vi "average fifo data.vi"(7 "Interleaved Data":i16[](array[numeric]), 17 "Samples":i32=1000, 18 "Acc":i32=200, 19 "error in (no error)":errorcluster) -> (6 "CD_signals":waveform(dbl), 8 "Avg Scan":dbl[](graph), 14 "error out (no error)":errorcluster)   [LabVIEW 2015, in "io runtime.lvclass"]
uses:
  io runtime.lvclass
  <vilib>/Analysis/NI_AALBase.lvlib
  <vilib>/Analysis/baseanly.llb/Mean (DBL).vi
panel:
  in  "Channels":i32=4
  out "Avg Scan+1":dbl[](graph)
  out "Low DC":dbl
  out "DC":dbl
  out "First 5000":i16[](graph)
  out "Process Time":u32
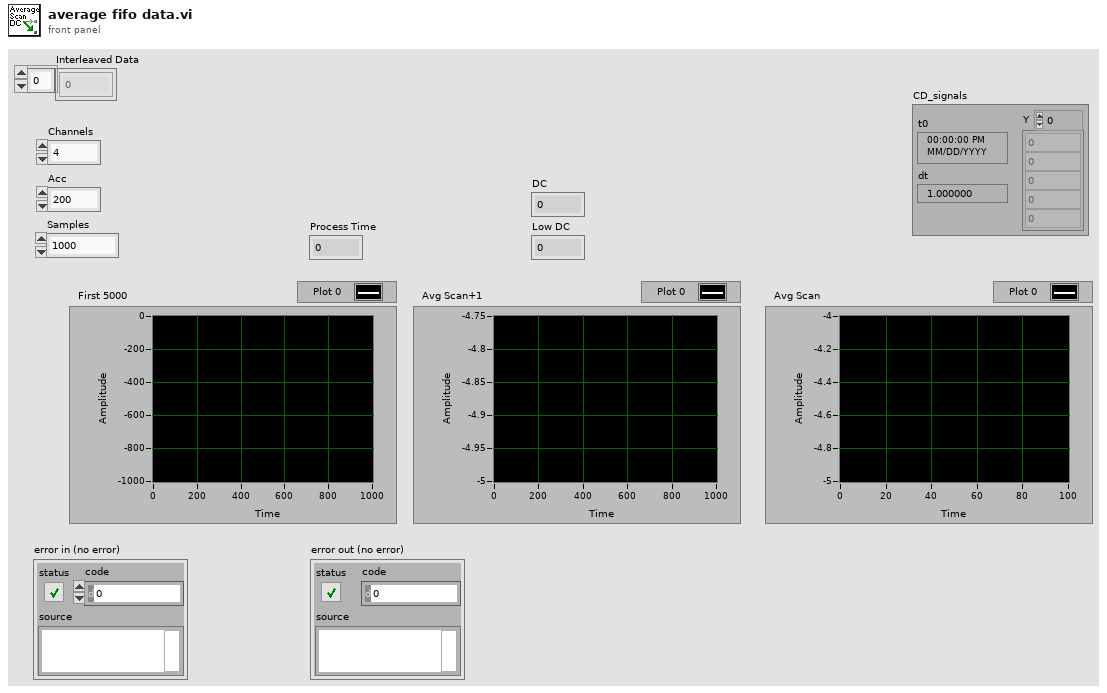
[diagram p1: front panel]
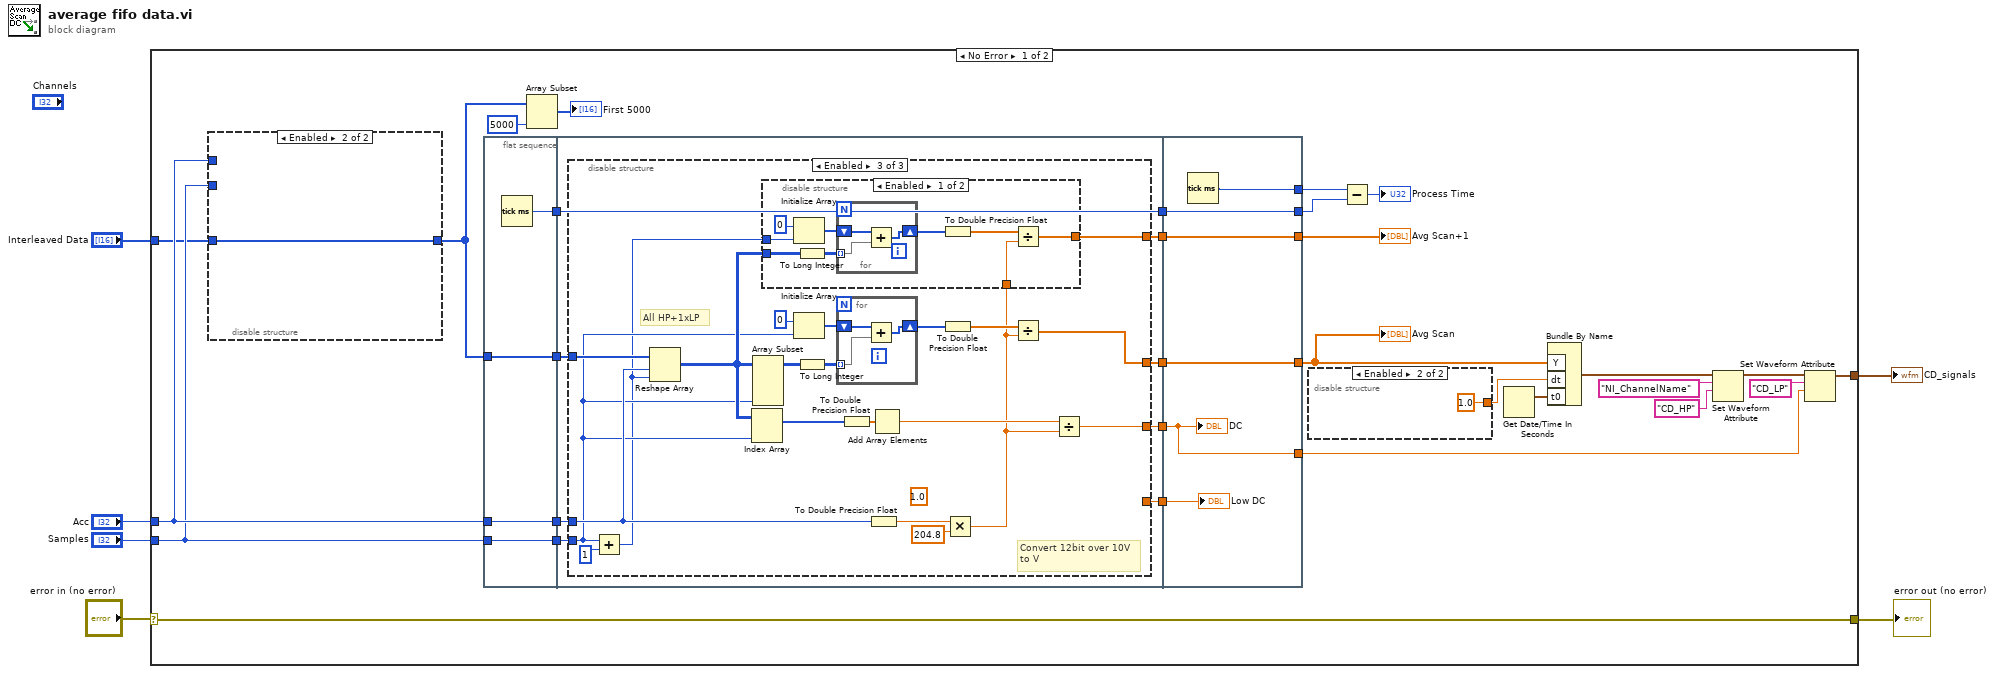
[diagram p0: block diagram]
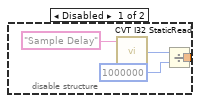
[diagram p2: hidden frame]
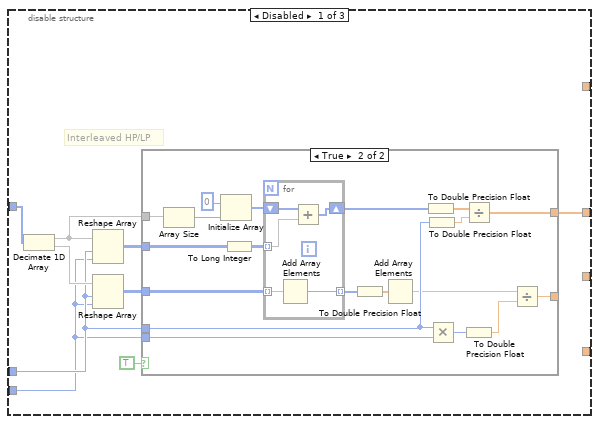
[diagram p3: hidden frame]
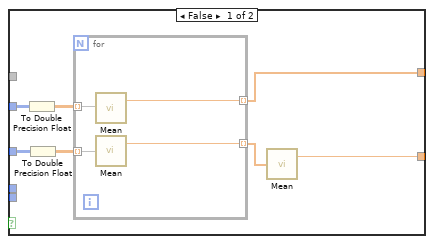
[diagram p4: hidden frame]
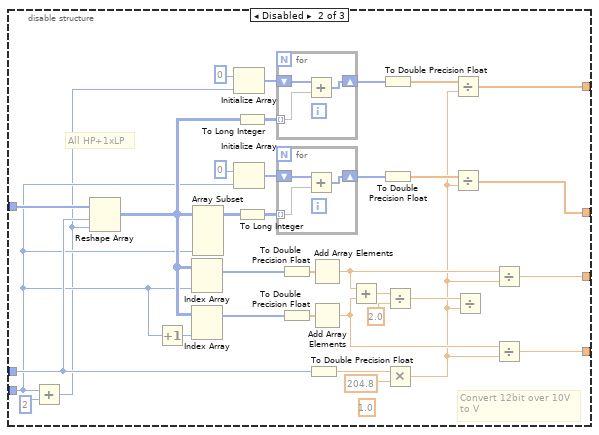
[diagram p5: hidden frame]
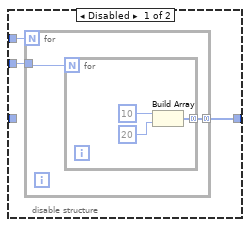
[diagram p7: hidden frame]
diagram:
  n1 = case shown="No Error" "error in (no error)" {
    selector: "error in (no error)" -> [w33 w189]
    tunnel: "Acc" -> [w36 _]
    tunnel: "Samples" -> [w35 _]
    tunnel: "Interleaved Data" -> [w34 _]
    tunnel: [w33 w189] -> w2
    tunnel: [w7 _] -> w1
    frame No Error {
      n2 = disable-structure shown="Enabled" {
        disable-tunnel: [w182 w188] -> w19
        disable-tunnel: w36 -> [w181 _]
        disable-tunnel: w35 -> [w180 _]
        disable-tunnel: w34 -> [_ w188]
        frame Disabled {
          n3 = for {
            N: w181 -> [_]
            tunnel: [w184] -> w182 mode=concatenating
            tunnel: w180 -> [w183]
            n4 = for {
              N: w183 -> [_]
              tunnel: [w185] -> w184 mode=concatenating
              n5 = Build Array(10, 20) -> (w185:i32[])
            }
          }
        }
        frame Enabled {
        }
      }
      n6 = flat-sequence {
        tunnel: w35 -> [w43]
        tunnel: w36 -> [w44]
        tunnel: w19 -> [w45]
        tunnel: [w45] -> w27
        tunnel: [w44] -> w26
        tunnel: [w43] -> w25
        tunnel: [w42] -> w20
        tunnel: w27 -> [w53]
        tunnel: w26 -> [w52]
        tunnel: w25 -> [w51]
        tunnel: [w50] -> w24
        tunnel: [w49] -> w21
        tunnel: w20 -> [w49]
        tunnel: [w48] -> w15
        tunnel: [w47] -> w14
        tunnel: [w46] -> w13
        tunnel: [w174] -> w8
        tunnel: [w175] -> w12
        tunnel: w24 -> [w175]
        tunnel: [w179] -> w22
        tunnel: [w178] -> w11
        tunnel: w21 -> [w178]
        tunnel: [w177] -> w16
        tunnel: w15 -> [w177]
        tunnel: w14 -> [w174]
        tunnel: w13 -> [w176]
        frame #0 {
          n7 = Tick Count (ms)() -> (millisecond timer value=w42:u32)
        }
        frame #1 {
          n8 = disable-structure shown="Enabled" {
            disable-tunnel: w53 -> [w58 w123 w150]
            disable-tunnel: w52 -> [w57 w122 w149]
            disable-tunnel: w51 -> [w56 w103 w142]
            disable-tunnel: [w55 w121 w148] -> w50
            disable-tunnel: [_ w104 w143] -> w48
            disable-tunnel: [_ w100 w140] -> w47
            disable-tunnel: [_ w99 _] -> w46
            frame Disabled {
              # "Interleaved HP/LP"
              n9 = Decimate 1D Array(w58) -> (w59:i16[], w62:i16[])
              n10 = Reshape Array(w59, w57, w56) -> (w61:i16[][])
              n11 = Reshape Array(w62, w57, w56) -> (w60:i16[][])
              n12 = case shown="True" TRUE {
                tunnel: w57 -> [_ w92]
                tunnel: w61 -> [w69 w91]
                tunnel: w60 -> [w68 w90]
                tunnel: w59 -> [_ w84]
                tunnel: [w63 w83] -> _
                tunnel: w56 -> [_ w77]
                tunnel: [w67 w76] -> w55
                frame False {
                  n13 = To Double Precision Float(number=w69) -> (double precision float=w66:dbl[][])
                  n14 = To Double Precision Float(number=w68) -> (double precision float=w65:dbl[][])
                  n15 = for {
                    tunnel: w66 -> [w73] mode=indexing
                    tunnel: w65 -> [w71] mode=indexing
                    tunnel: [w72] -> w67 mode=indexing
                    tunnel: [w70] -> w64 mode=indexing
                    n16 = call-poly <vilib>:"Mean.vi"("X"=w73) -> ("mean"=w72:dbl)  [unwired: 1 out]
                    n17 = call-poly <vilib>:"Mean.vi"("X"=w71) -> ("mean"=w70:dbl)  [unwired: 1 out]
                  }
                  n18 = call-poly <vilib>:"Mean.vi"("X"=w64) -> ("mean"=w63:dbl)  [unwired: 1 out]
                }
                frame True {
                  n19 = Array Size(array=w84) -> (size(s)=w85:i32)
                  n20 = Initialize Array(0, w85) -> (w87:i32[])
                  n21 = To Long Integer(number=w91) -> (32bit integer=w78:i32[][])
                  n22 = for {
                    tunnel: w78 -> [w96] mode=indexing
                    shift-right: [w97] -> w89
                    shift-left: w87 -> [w95]
                    tunnel: w90 -> [w94] mode=indexing
                    tunnel: [w93] -> w81 mode=indexing
                    n23 = Add Array Elements(numeric array=w94) -> (sum=w93:i16)
                    n24 = Add(x=w95, y=w96) -> (x+y=w97:i32[])
                  }
                  n25 = To Double Precision Float(number=w81) -> (double precision float=w80:dbl[])
                  n26 = Add Array Elements(numeric array=w80) -> (sum=w79:dbl)
                  n27 = To Double Precision Float(number=w89) -> (double precision float=w88:dbl[])
                  n28 = To Double Precision Float(number=w92) -> (double precision float=w82:dbl)
                  n29 = Multiply(x=w92, y=w77) -> (x*y=w75:i32)
                  n30 = Divide(x=w88, y=w82) -> (x/y=w76:dbl[])
                  n31 = To Double Precision Float(number=w75) -> (double precision float=w74:dbl)
                  n32 = Divide(x=w79, y=w74) -> (x/y=w83:dbl)
                }
              }
            }
            frame Disabled {
              (unwired) 1.0 ("y")
              # "Convert 12bit over 10V\nto V"
              # "All HP+1xLP"
              n33 = Add(x=w103, y=2) -> (x+y=w102:i32)
              n34 = Reshape Array(w123, w122, w102) -> (w106:i16[][])
              n35 = Increment(x=w103) -> (x+1=w114:i32)
              n36 = Index Array(array=w106, index (col)=w103) -> (element=w124:i16[])  [unwired: 1 in]
              n37 = Index Array(array=w106, index (col)=w114) -> (element=w119:i16[])  [unwired: 1 in]
              n38 = Array Subset(array=w106, length (col)=w103) -> (w125:i16[][])  [unwired: 3 in]
              n39 = Initialize Array(0, w102) -> (w108:i32[])
              n40 = Initialize Array(0, w103) -> (w129:i32[])
              n41 = To Long Integer(number=w106) -> (32bit integer=w110:i32[][])
              n42 = To Long Integer(number=w125) -> (32bit integer=w126:i32[][])
              n43 = for {
                tunnel: w110 -> [w133] mode=indexing
                shift-right: [w134] -> w107
                shift-left: w108 -> [w132]
                n44 = Add(x=w132, y=w133) -> (x+y=w134:i32[])
              }
              n45 = for {
                tunnel: w126 -> [w136] mode=indexing
                shift-right: [w137] -> w131
                shift-left: w129 -> [w135]
                n46 = Add(x=w135, y=w136) -> (x+y=w137:i32[])
              }
              n47 = To Double Precision Float(number=w124) -> (double precision float=w127:dbl[])
              n48 = To Double Precision Float(number=w119) -> (double precision float=w120:dbl[])
              n49 = To Double Precision Float(number=w122) -> (double precision float=w118:dbl)
              n50 = Add Array Elements(numeric array=w127) -> (sum=w112:dbl)
              n51 = Add Array Elements(numeric array=w120) -> (sum=w111:dbl)
              n52 = Add(x=w112, y=w111) -> (x+y=w117:dbl)
              n53 = To Double Precision Float(number=w107) -> (double precision float=w105:dbl[])
              n54 = To Double Precision Float(number=w131) -> (double precision float=w130:dbl[])
              n55 = Divide(x=w117, y=2.0) -> (x/y=w113:dbl)
              n56 = Multiply(x=w118, y=204.8) -> (x*y=w101:dbl)
              n57 = Divide(x=w105, y=w101) -> (x/y=w104:dbl[])
              n58 = Divide(x=w130, y=w101) -> (x/y=w121:dbl[])
              n59 = Divide(x=w113, y=w101) -> ()  [unwired: 1 out]
              n60 = Divide(x=w112, y=w101) -> (x/y=w100:dbl)
              n61 = Divide(x=w111, y=w101) -> (x/y=w99:dbl)
            }
            frame Enabled {
              (unwired) 1.0 ("y")
              # "Convert 12bit over 10V\nto V"
              # "All HP+1xLP"
              n62 = Add(x=w142, y=1) -> (x+y=w141:i32)
              n63 = Reshape Array(w150, w149, w141) -> (w144:i16[][])
              n64 = Index Array(array=w144, index (col)=w142) -> (element=w151:i16[])  [unwired: 1 in]
              n65 = Array Subset(array=w144, length (col)=w142) -> (w152:i16[][])  [unwired: 3 in]
              n66 = Initialize Array(0, w142) -> (w156:i32[])
              n67 = To Long Integer(number=w152) -> (32bit integer=w153:i32[][])
              n68 = for {
                tunnel: w153 -> [w172] mode=indexing
                shift-right: [w173] -> w158
                shift-left: w156 -> [w171]
                n69 = Add(x=w171, y=w172) -> (x+y=w173:i32[])
              }
              n70 = To Double Precision Float(number=w151) -> (double precision float=w154:dbl[])
              n71 = To Double Precision Float(number=w149) -> (double precision float=w147:dbl)
              n72 = Add Array Elements(numeric array=w154) -> (sum=w145:dbl)
              n73 = To Double Precision Float(number=w158) -> (double precision float=w157:dbl[])
              n74 = Multiply(x=w147, y=204.8) -> (x*y=w139:dbl)
              n75 = disable-structure shown="Enabled" {
                disable-tunnel: w144 -> [w163 _]
                disable-tunnel: [w161 _] -> w143
                disable-tunnel: w141 -> [w160 _]
                disable-tunnel: w139 -> [w159 _]
                frame Enabled {
                  n76 = Initialize Array(0, w160) -> (w165:i32[])
                  n77 = To Long Integer(number=w163) -> (32bit integer=w167:i32[][])
                  n78 = for {
                    tunnel: w167 -> [w169] mode=indexing
                    shift-right: [w170] -> w164
                    shift-left: w165 -> [w168]
                    n79 = Add(x=w168, y=w169) -> (x+y=w170:i32[])
                  }
                  n80 = To Double Precision Float(number=w164) -> (double precision float=w162:dbl[])
                  n81 = Divide(x=w162, y=w159) -> (x/y=w161:dbl[])
                }
                frame Disabled {
                }
              }
              n82 = Divide(x=w157, y=w139) -> (x/y=w148:dbl[])
              n83 = Divide(x=w145, y=w139) -> (x/y=w140:dbl)
            }
          }
        }
        frame #2 {
          n84 = Tick Count (ms)() -> (millisecond timer value=w179:u32)
          "DC" <- w174
          "Low DC" <- w176
        }
      }
      n85 = Array Subset(array=w19, length=5000) -> (→"First 5000":i16[])  [unwired: 1 in]
      n86 = disable-structure shown="Enabled" {
        disable-tunnel: [w40 1.0] -> w32
        frame Disabled {
          n87 = call <vilib>:"CVT I32 StaticRead.vi"("Tag Name"="Sample Delay") -> ("Value"=w38:i32)  [unwired: 3 in, 1 out]
          n88 = Divide(x=w38, y=1000000) -> (x/y=w40:dbl)
        }
        frame Enabled {
        }
      }
      n89 = Subtract(x=w22, y=w11) -> (x-y=→"Process Time":u32)
      n90 = Get Date/Time In Seconds() -> (seconds since 1Jan1904=w28:timestamp)
      n91 = Bundle By Name("Y"=w12, "dt"=w32, "t0"=w28) -> (w29:waveform(dbl))  [unwired: 1 in]
      n92 = Set Waveform Attribute(5:"CD_HP" ("name"), 6:"NI_ChannelName" ("name"), 7:w29) -> (3:w9:waveform(dbl))  [unwired: 1 in, 2 out]
      n93 = Set Waveform Attribute(5:w8, 6:"CD_LP" ("name"), 7:w9) -> (3:w7:waveform(dbl))  [unwired: 1 in, 2 out]
      "Avg Scan" <- w12
      "Avg Scan+1" <- w16
    }
    frame Error {
    }
  }
  "error out (no error)" <- w2
  "CD_signals" <- w1
